vi "Config Base Path Init.vi"(8 "error in":errorcluster, 10 "TS Name":string, 11 "base path":path) -> (0 "error out":errorcluster, 3 "TS Config Folder Path":path)   [LabVIEW 2019, in "Generic Test Stand.lvclass"]
doc: "Return path to folder inside project base directory. If folder does not exist - create it."
uses:
  Generic Test Stand.lvclass
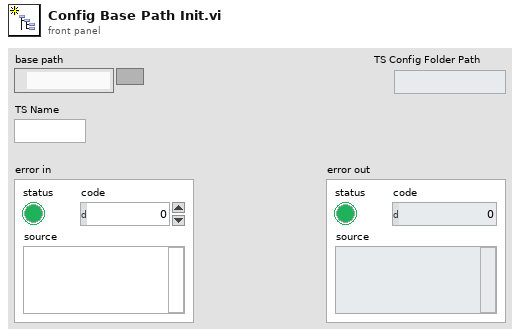
[diagram p1: front panel]
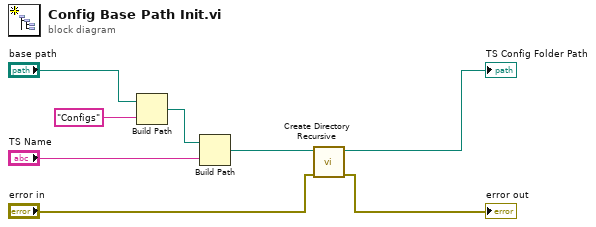
[diagram p0: block diagram]
diagram:
  n1 = Build Path(base path="base path", name or relative path="Configs") -> (appended path=w6:path)
  n2 = Build Path(base path=w6, name or relative path="TS Name") -> (appended path=w4:path)
  n3 = call <vilib>:"Create Directory Recursive.vi"("error in (no error)"="error in", "directory"=w4) -> ("error out"=→"error out":errorcluster, "directory copy"=→"TS Config Folder Path":path)  [unwired: 3 in, 1 out]
